vi "11e-async.vi"() -> ()   [LabVIEW 2018, in "LV2Julia_examples.lvlib"]
uses:
  LV2Julia_examples.lvlib
  LV2Julia_core/VIs/Server or client state.ctl
  LV2Julia_core/VIs/detailed error info.ctl
  LV2Julia_core/VIs/StackFrame.ctl
  LV2Julia_core/VIs/Commands.ctl
  LV2Julia_core/VIs/polling control.ctl
  48781df3-20eb-4f5d-8082-2d6b3742813b.vi
  48781df3-20eb-4f5d-8082-2d6b3742813b.vi/7dc80a6f-5b72-4e6e-b30f-f7177a9c8dda.vi
  48781df3-20eb-4f5d-8082-2d6b3742813b.vi/7dc80a6f-5b72-4e6e-b30f-f7177a9c8dda.vi/d1582522-19a1-4d14-9751-f201deff1c68.vi
  48781df3-20eb-4f5d-8082-2d6b3742813b.vi/7dc80a6f-5b72-4e6e-b30f-f7177a9c8dda.vi/d1582522-19a1-4d14-9751-f201deff1c68.vi/1fe1509c-f277-4f5e-9152-f85924663264.vi
  48781df3-20eb-4f5d-8082-2d6b3742813b.vi/7dc80a6f-5b72-4e6e-b30f-f7177a9c8dda.vi/d1582522-19a1-4d14-9751-f201deff1c68.vi/a9b676c7-50e6-4ffc-bed7-bb5ff5be4752.vi
  48781df3-20eb-4f5d-8082-2d6b3742813b.vi/7dc80a6f-5b72-4e6e-b30f-f7177a9c8dda.vi/d1582522-19a1-4d14-9751-f201deff1c68.vi/1d182be8-62d3-4883-b855-b672dc84849d.vi
  LV2Julia_core/VIs/jl-scripts path.vi
  LV2Julia_core/VIs/check ID validity.vi
  LV2Julia_core/VIs/bindata_descr to JSON.vi
  LV2Julia_core/VIs/check cluster field names.vi
  LV2Julia_core/VIs/concat JSON.vi
  LV2Julia_core/VIs/build request.vi
  LV2Julia_core/VIs/Parse server response.vi
  LV2Julia_core/VIs/log jl exceptions.vi
  LV2Julia_core/VIs/poll spawned task.vi
  LV2Julia_core/LV2Julia_core.lvlib
panel:
  in  "Timeout (s)":dbl=-1.0
  out "notification":bool
  in  "stop polling":bool
  out "stopping":bool
  out "done":bool
  in  "summands":cluster{"x":dbl, "y":dbl}={"x"=2.0, "y"=2.0}
  in  "next":bool
  out "x+y":dbl=nan
  out "detailed error info":T1
  out "current error":errorcluster
  out "final error":errorcluster
  out "short err code":u8
  in  "stop":bool
  out "ZMQ timeout":bool
  out "Julia script file path":path
  out "temporary script path":path
  out "Jl Server state":T3
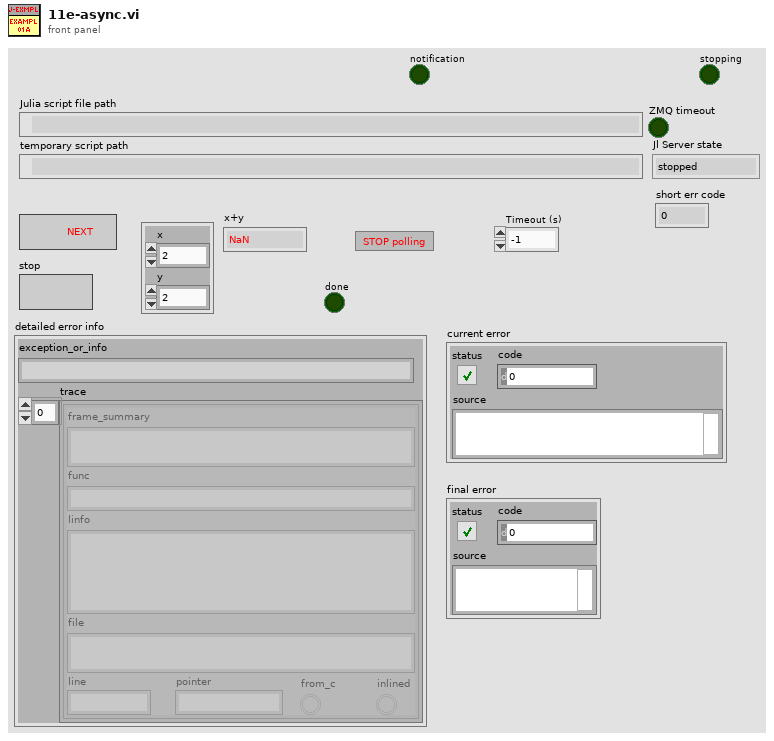
[diagram p1: front panel]
types:
  T1 = typedef "LV2Julia_core.lvlib/detailed error info.ctl" = cluster{"exception_or_info":string, "trace":T2[]}
  T2 = typedef "LV2Julia_core.lvlib/StackFrame.ctl" = cluster{"frame_summary":string, "func":string, "linfo":string, "file":string, "line":i32, "pointer":u64, "from_c":bool, "inlined":bool}
  T3 = typedef "LV2Julia_core.lvlib/Server or client state.ctl" = enum16{"stopped", "running", "unknown"}
  T4 = typedef "LV2Julia_core.lvlib/Commands.ctl" = enum16{"Start Jl-server & Init LV-client", "Send request & Get response ", "Stop Jl-server & Cleanup LV-client", "Cleanup LV-client", "Start Jl-server", "Stop Jl-server", "Init LV-Client", "Cleanup LV-Client", "(not allowed)", "Set LV Client state", "Set Jl Server state", "set ZMQ timeout", "read ZMQ timeout", "read-out state"}
  T5 = typedef "Server state info.ctl" = cluster{"detailed error info":T1, "return code":u8, "Jl Server state":T3}
  T6 = typedef "LV2Julia_core.lvlib/polling control.ctl" = cluster{"Timeout, ms (-1)":i32, "polling period (ms)":cluster{"starting":i32, "final":i32}, "interrupt polling notifier":refnum<notifier>}
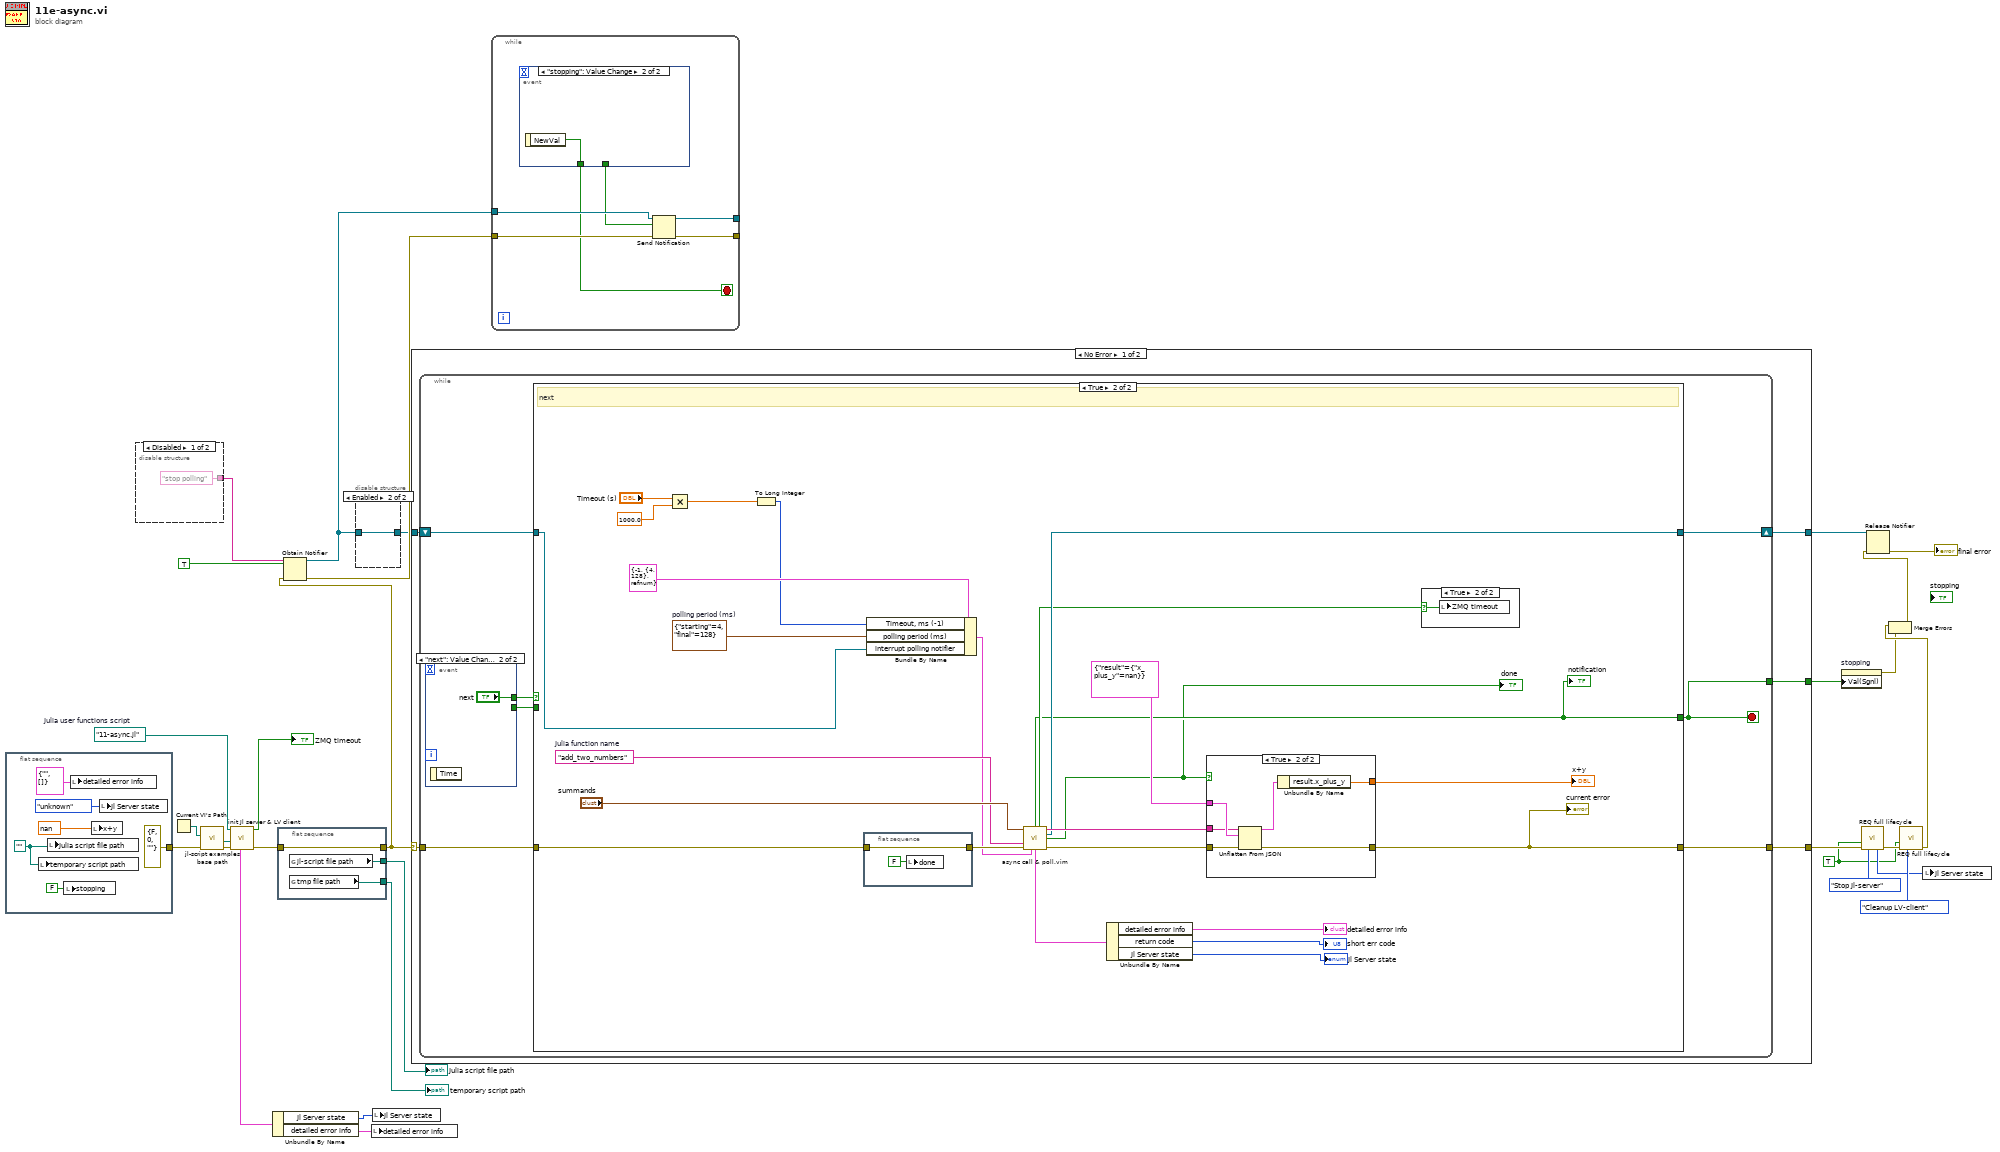
[diagram p0: block diagram]
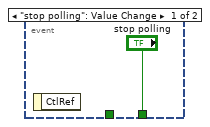
[diagram p4: hidden frame]
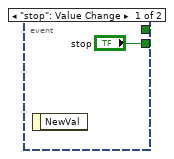
[diagram p5: hidden frame]
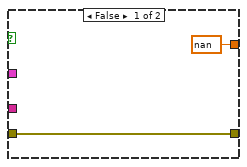
[diagram p7: hidden frame]
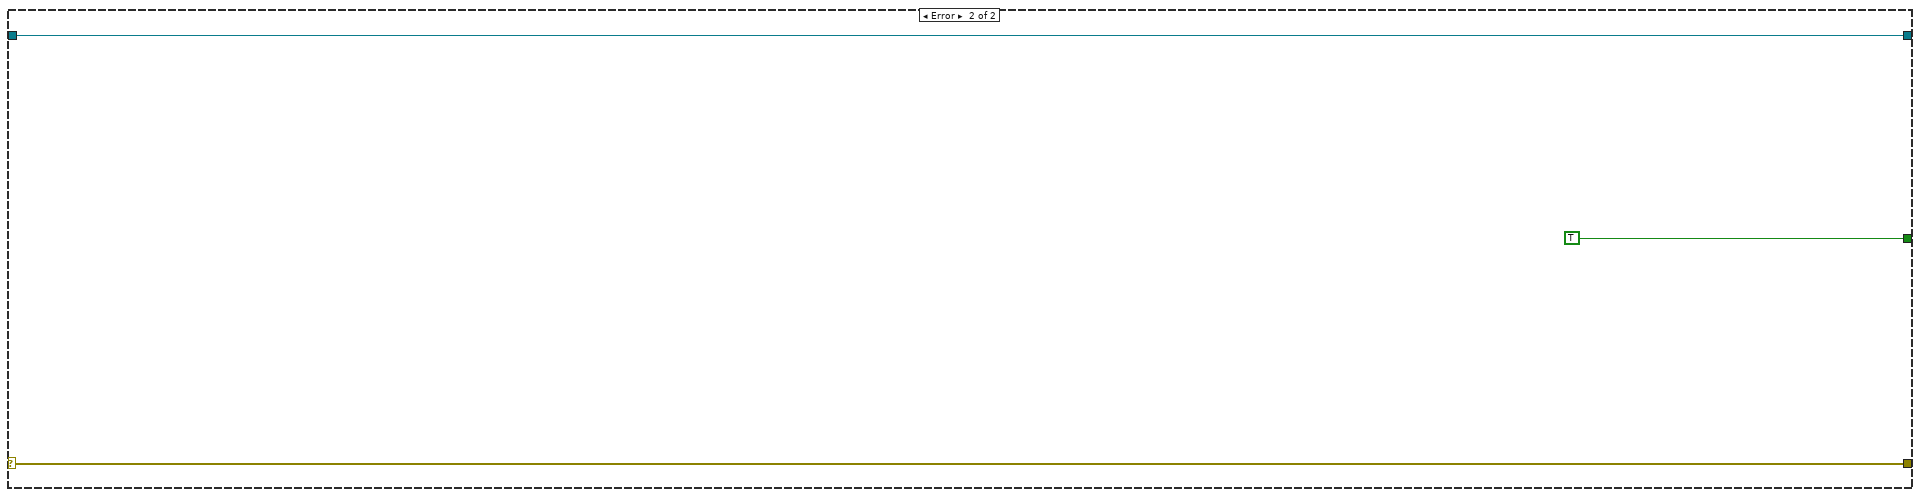
[diagram p9: hidden frame]
diagram:
  w23 = path "11-async.jl"  # Julia user functions script
  w9 = TRUE ("Force command")
  n1 = flat-sequence {
    tunnel: [errorcluster {"status"=FALSE, "code"=0, "source"=""} ("error in (no error)")] -> w20
    frame #0 {
      w32 = path ""
      n2 = local write "temporary script path"(w32) -> ()
      n3 = local write "Julia script file path"(w32) -> ()
      n4 = local write "stopping"(FALSE ("stopping")) -> ()
      n5 = local write "detailed error info"(T1 {"exception_or_info"="", "trace"=[]} ("detailed error info")) -> ()
      n6 = local write "x+y"(nan ("Server response")) -> ()
      n7 = local write "Jl Server state"(Server_or_client_state."unknown" ("Jl Server state out")) -> ()
    }
  }
  n8 = disable-structure shown="Disabled" {
    disable-tunnel: ["stop polling" ("name (unnamed)") _] -> w14
    frame Disabled {
    }
    frame Enabled {
    }
  }
  n9 = Current VI's Path() -> (path=w17:path)
  n10 = call "jl-script examples base path.vi"("error in (no error)"=w20, "calling example VI path"=w17) -> ("error out"=w19:errorcluster, "jl-script-examples base path"=w18:path)  [unwired: 8 in]
  n11 = call "init Jl server & LV client.vi"("error in (no error)"=w19, "Base path (not a path)"=w18, "Julia user functions script"=w23) -> ("error out"=w21:errorcluster, "timeout?"=→"ZMQ timeout":bool, "Server state info"=w16:T5)  [unwired: 5 in, 1 out]
  n12 = Unbundle By Name(w16) -> ("Jl Server state"=w1:T3, "detailed error info"=w2:T1)
  n13 = flat-sequence {
    tunnel: [w40] -> w13
    tunnel: w21 -> [w40]
    tunnel: [w39] -> w25
    tunnel: [w38] -> w26
    frame #0 {
      n14 = global read "jl-scripts path.vi" "jl-script file path"() -> (w39:path)
      n15 = global read "jl-scripts path.vi" "tmp file path"() -> (w38:path)
    }
  }
  n16 = Obtain Notifier(name (unnamed)=w14, notification data type=TRUE, error in (no error)=w13) -> (notifier out=w3:refnum<notifier>, error out=w12:errorcluster)  [unwired: 1 in, 1 out]
  n17 = disable-structure shown="Enabled" {
    disable-tunnel: [_ w41] -> w4
    disable-tunnel: w3 -> [_ w41]
    frame Disabled {
    }
    frame Enabled {
    }
  }
  n18 = local write "detailed error info"(w2) -> ()
  n19 = local write "Jl Server state"(w1) -> ()
  n20 = case shown="No Error" w13 {
    selector: w13 -> [w45 w97]
    tunnel: [w46 w97] -> w30
    tunnel: w4 -> [w44 w96]
    tunnel: [w43 w96] -> w11
    tunnel: [w42 TRUE ("stop")] -> w5
    frame No Error {
      n21 = while {
        tunnel: w45 -> [w52]
        tunnel: [w53] -> w46
        shift-right: [w48] -> w43
        shift-left: w44 -> [w49]
        tunnel: [w47] -> w42
        stop <- w47 stop-if-true
        n22 = event shown="[1] \"next\": Value Change" {
          selector: _ -> [_ _]
          dyn-events: _ -> [_ _]
          timeout: _ -> [_ _]
          tunnel: [_ "next"] -> w51
          tunnel: ["stop" _] -> w50
          event "stop": Value Change {
            n23 = event-data() -> ()  [unwired: 1 in, 1 out]
          }
          event "next": Value Change {
            n24 = event-data() -> ()  [unwired: 1 in, 1 out]
          }
        }
        n25 = case shown="True" w51 {
          tunnel: [w56 w82] -> w53
          tunnel: w52 -> [w56 w65]
          tunnel: [w57 w67] -> w47
          tunnel: w50 -> [w57 _]
          tunnel: w49 -> [w58 w73]
          tunnel: [w58 w69] -> w48
          frame False {
            # "stop"
          }
          frame True {
            w74 = cluster{"starting":i32, "final":i32} {"starting"=4, "final"=128}  # polling period (ms)
            w71 = "add_two_numbers"  # Julia function name
            # "next"
            n26 = Multiply(x="Timeout (s)", y=1000.0) -> (x*y=w77:dbl)
            n27 = To Long Integer(number=w77) -> (32bit integer=w75:i32)
            n28 = flat-sequence {
              tunnel: [w85] -> w64
              tunnel: w65 -> [w85]
              frame #0 {
                n29 = local write "done"(FALSE ("done")) -> ()
              }
            }
            n30 = Bundle By Name(cluster=T6 {"Timeout, ms (-1)"=-1, "polling period (ms)"={"starting"=4, "final"=128}, "interrupt polling notifier"=refnum} ("polling control"), "Timeout, ms (-1)"=w75, "polling period (ms)"=w74, "interrupt polling notifier"=w73) -> (w62:T6)
            n31 = call "async call & poll.vim"("Arguments 1"="summands", "Julia function name"=w71, "error in (no error)"=w64, "polling control"=w62) -> ("Notification out"=w67:bool, "timeout?"=w68:bool, "JSON received"=w70:string, "Notifier out"=w69:refnum<notifier>, "done"=w66:bool, "Server state info"=w63:T5, "error out"=w81:errorcluster)  [unwired: 5 in]
            "done" <- w66
            "notification" <- w67
            n32 = Unbundle By Name(w63) -> ("detailed error info"=→"detailed error info":T1, "return code"=→"short err code":u8, "Jl Server state"=→"Jl Server state":T3)
            n33 = case shown="True" w66 {
              tunnel: [nan ("x_plus_y") w93] -> w83
              tunnel: [w87 w91] -> w82
              tunnel: w81 -> [w87 w90]
              tunnel: cluster{"result":cluster{"x_plus_y":dbl}} {"result"={"x_plus_y"=nan}} -> [_ w89]
              tunnel: w70 -> [_ w88]
              frame False {
              }
              frame True {
                n34 = Unflatten From JSON(JSON string=w88, type and defaults=w89, error in (no error)=w90) -> (value=w92:cluster{"result":cluster{"x_plus_y":dbl}}, error out=w91:errorcluster)  [unwired: 4 in]
                n35 = Unbundle By Name(w92) -> ("result.x_plus_y"=w93:dbl)
              }
            }
            "current error" <- w82
            "x+y" <- w83
            n36 = case shown="True" w68 {
              selector: w68 -> [_ w94]
              frame False {
              }
              frame True {
                n37 = local write "ZMQ timeout"(w94) -> ()
              }
            }
          }
        }
      }
    }
    frame Error {
    }
  }
  n38 = while {
    tunnel: w3 -> [w103]
    tunnel: [w102] -> _
    tunnel: w12 -> [w101]
    tunnel: [w100] -> _
    stop <- w98 stop-if-true
    n39 = event shown="[1] \"stopping\": Value Change" {
      selector: _ -> [_ _]
      dyn-events: _ -> [_ _]
      timeout: _ -> [_ _]
      tunnel: ["stop polling" _] -> w99
      tunnel: [_ w105] -> w98
      event "stop polling": Value Change {
        n40 = event-data() -> ()  [unwired: 1 in, 1 out]
      }
      event "stopping": Value Change {
        n41 = event-data() -> ("NewVal"=w105:bool)  [unwired: 1 in]
      }
    }
    n42 = Send Notification(notification=w99, notifier=w103, error in (no error)=w101) -> (notifier out=w102:refnum<notifier>, error out=w100:errorcluster)
  }
  n43 = property on="stopping" class="Bool (strict)"("Val(Sgnl)"=w5) -> (error out=w6:errorcluster)  [unwired: 2 in, 1 out]
  n44 = call "REQ full lifecycle.vi"("Force command"=w9, "error in"=w30, "command"=Commands."Stop Jl-server") -> ("Jl Server state out"=w24:T3, "error out"=w28:errorcluster)  [unwired: 6 in, 5 out]
  n45 = call "REQ full lifecycle.vi"("Force command"=w9, "error in"=w28, "command"=Commands."Cleanup LV-client") -> ("error out"=w8:errorcluster)  [unwired: 6 in, 6 out]
  n46 = Merge Errors(w8, w6) -> (w7:errorcluster)
  n47 = Release Notifier(notifier=w11, error in (no error)=w7) -> (error out=→"final error":errorcluster)  [unwired: 1 in, 2 out]
  n48 = local write "Jl Server state"(w24) -> ()
  "temporary script path" <- w26
  "Julia script file path" <- w25
